vi "Axis_Editor.vi"() -> ()   [LabVIEW 2012]
panel:
  in  "CancelButton":bool
  in  "OKButton":bool
  in  "Grids":bool caption="Show Grids"
  in  "Auto":bool caption="Auto?"
  in  "Incr":dbl caption="Label Increment:"
  in  "MinVal":dbl caption="Minimum Value:"
  in  "MaxVal":dbl caption="Maximum Value:"
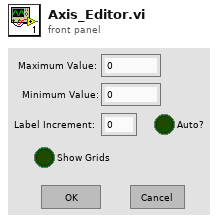
[diagram p1: front panel]
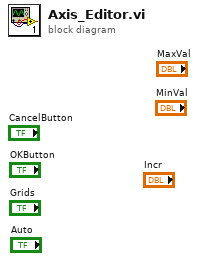
[diagram p0: block diagram]
diagram:
